vi "Read Conveyor.vi"(8 "error in (no error)":errorcluster, 11 "ODESimulator_Base_Conveyor in":refnum<class "ODESimulator_Base_Conveyor.lvclass">) -> (0 "error out":errorcluster, 2 "Conveyor":refnum<k20>, 3 "ODESimulator_Base_Conveyor out":refnum<class "ODESimulator_Base_Conveyor.lvclass">)   [LabVIEW 2017, in "NI_Robotics_Simulator.lvlib" / "ODESimulator_Base_Conveyor.lvclass"]
uses:
  <vilib>/robotics/Simulator/Robot Factory/Conveyor/Base/ODESimulator_Base_Conveyor.lvclass
  <vilib>/robotics/Simulator/Robot Factory/Conveyor/Base/ODESimulator_Base_Conveyor.lvclass/ODESimulator_Base_Conveyor.ctl
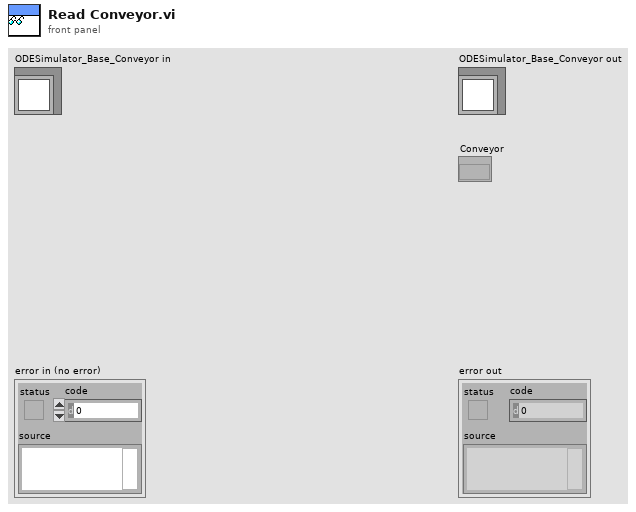
[diagram p1: front panel]
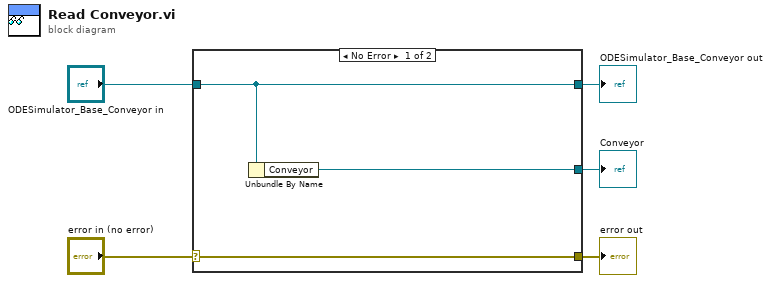
[diagram p0: block diagram]
diagram:
  n1 = case shown="No Error" "error in (no error)" {
    selector: "error in (no error)" -> [w8 w9]
    tunnel: [w8 w9] -> w4
    tunnel: [w7 w10] -> w2
    tunnel: "ODESimulator_Base_Conveyor in" -> [w7 w10]
    tunnel: [w6 _] -> w1
    frame No Error {
      n2 = Unbundle By Name(w7) -> ("Conveyor"=w6:refnum<k20>)
    }
    frame Error {
    }
  }
  "error out" <- w4
  "ODESimulator_Base_Conveyor out" <- w2
  "Conveyor" <- w1
